vi "GetPoseAndTargeting.vi"() -> ()   [LabVIEW 2019]
uses:
  refnums.vi
  GRNF_GenericMotor.vi
  dsinstructions.vi
  sensors.vi
  autoninfo.vi
  dsdata.vi
panel:
  out "Y Position (in)":dbl=94.7
  out "X Position (in)":dbl=509.2
  out "Heading (deg)":dbl format="%#_13g"
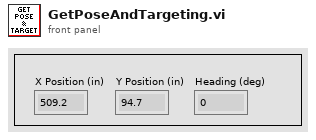
[diagram p1: front panel]
types:
  T1 = enum16{"Center", "North", "NorthWest", "West", "SouthWest", "South", "SouthEast", "East", "NorthEast"}
  T2 = typedef "WPI_MotorControlDeviceRef.ctl" = cluster{"DeviceStatus":errorcluster, "Type":T3, "PWM":cluster{"PWM Channel":T4, "DeadBand":T5}, "CAN":cluster{"Device Number":u8, "SetOutput VI Ref":variant, "GetOutput VI Ref":variant, "Enable VI Ref":variant, "Disable VI Ref":variant, "Data":variant}, "Invert":bool, "DIO PWM":cluster{"PWM \"Enable\" Channel":T4, "DIOChannel":T6, "PWM Rate":dbl}}
  T3 = typedef "WPI_MotorControlType.ctl" = enum16{"PWM", "CAN", "DIO PWM"}
  T4 = typedef "FPGA_DIOPWMChannel.ctl" = enum8{"PWM 0", "PWM 1", "PWM 2", "PWM 3", "PWM 4", "PWM 5", "PWM 6", "PWM 7", "PWM 8", "PWM 9", "PWM MXP 0", "PWM MXP 1", "PWM MXP 2", "PWM MXP 3", "PWM MXP 4", "PWM MXP 5", "PWM MXP 6", "PWM MXP 7", "PWM MXP 8", "PWM MXP 9", "Invalid"}
  T5 = typedef "WPI_PWMDeadband.ctl" = cluster{"Name":string, "maxPositivePwm":i32, "minPositivePwm":i32, "centerPwm":i32, "maxNegativePwm":i32, "minNegativePwm":i32, "angularRange":u16}
  T6 = typedef "FPGA_DIOChannel.ctl" = enum8{"DIO 0", "DIO 1", "DIO 2", "DIO 3", "DIO 4", "DIO 5", "DIO 6", "DIO 7", "DIO 8", "DIO 9", "DIO MXP 0", "DIO MXP 1", "DIO MXP 2", "DIO MXP 3", "DIO MXP 4", "DIO MXP 5", "DIO MXP 6", "DIO MXP 7", "DIO MXP 8", "DIO MXP 9", "DIO MXP 10", "DIO MXP 11", "DIO MXP 12", "DIO MXP 13", "DIO MXP 14", "DIO MXP 15", "SPI Port CS1", "SPI Port CS2", "SPI Port CS3", "SPI Port MISO", "SPI Port MOSI", "Invalid"}
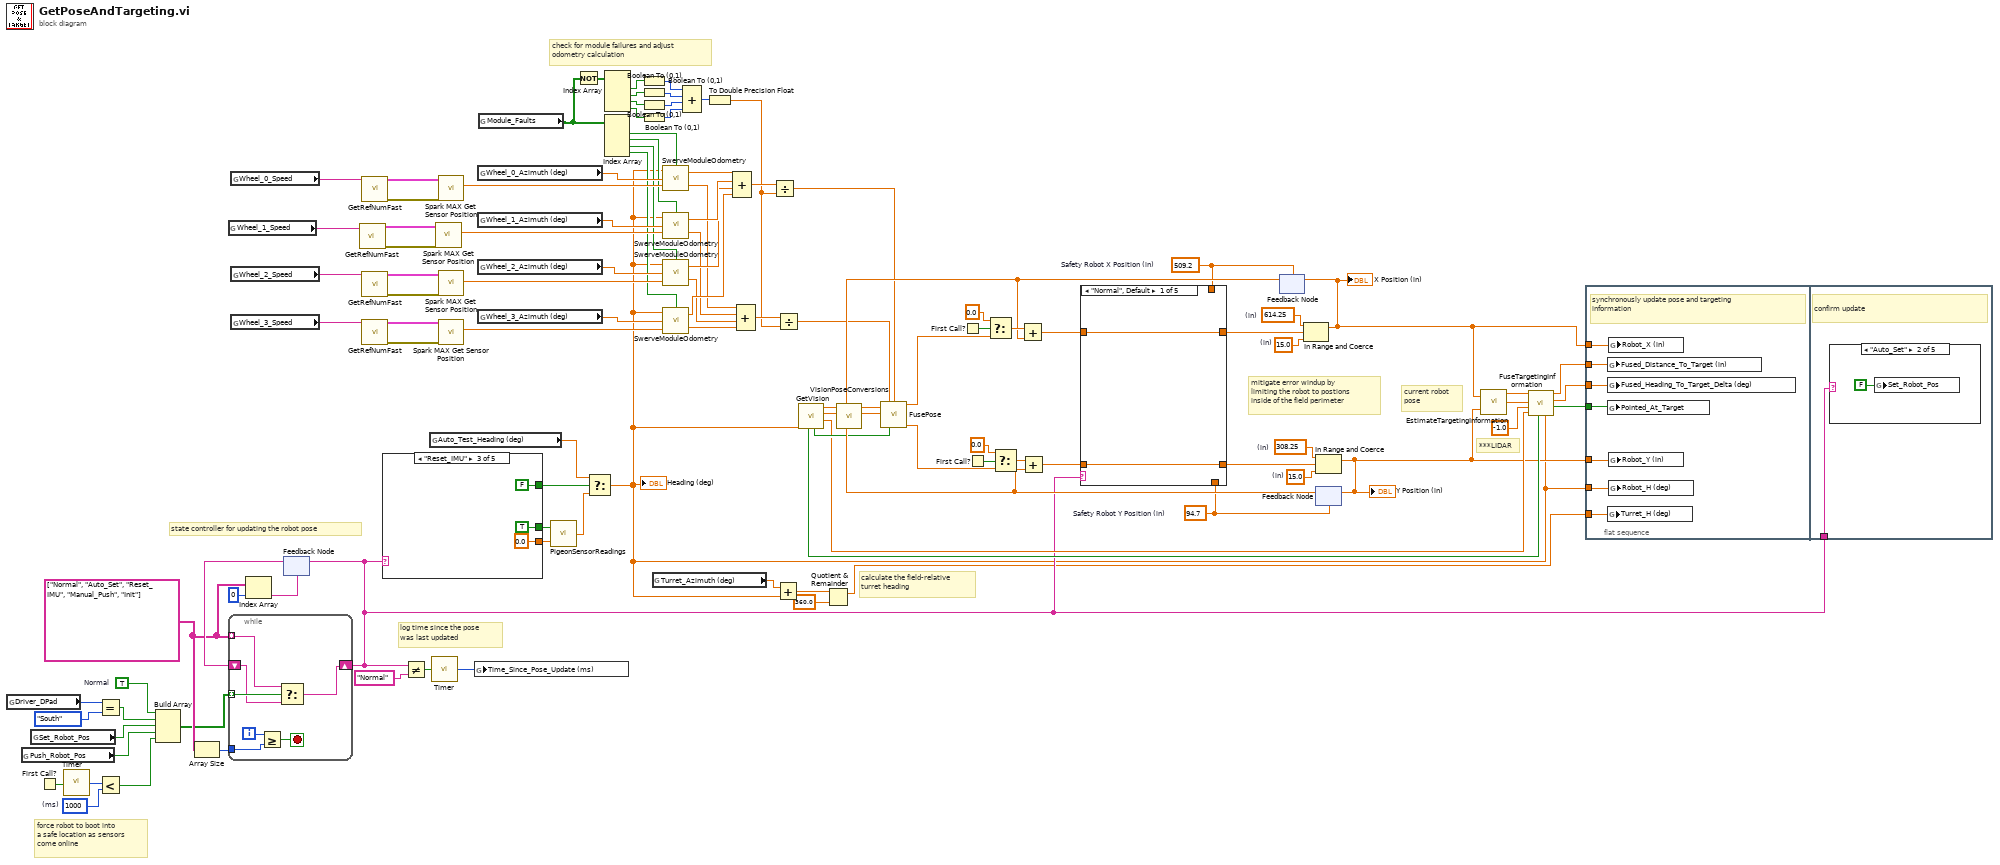
[diagram p0: block diagram]
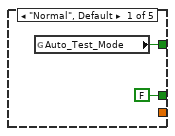
[diagram p6: hidden frame]
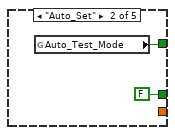
[diagram p7: hidden frame]
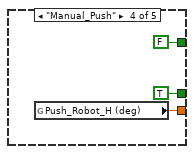
[diagram p8: hidden frame]
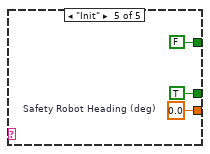
[diagram p9: hidden frame]
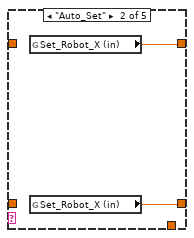
[diagram p10: hidden frame]
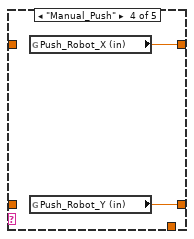
[diagram p12: hidden frame]
diagram:
  w2 = u32 1000  # (ms)
  w33 = string[] ["Normal", "Auto_Set", "Reset_IMU", "Manual_Push", "Init"] ("State Names")
  w32 = TRUE  # Normal
  w57 = 308.25  # (in)
  w58 = 15.0  # (in)
  w62 = 614.25  # (in)
  w63 = 15.0  # (in)
  w7 = 509.2  # Safety Robot X Position (in)
  w6 = 94.7  # Safety Robot Y Position (in)
  # "***LIDAR"
  # "force robot to boot into\na safe location as sensors\ncome online"
  # "calculate the field-relative\nturret heading"
  # "log time since the pose\nwas last updated"
  # "state controller for updating the robot pose"
  # "current robot\npose"
  # "mitigate error windup by\nlimiting the robot to postions\ninside of the field perimeter"
  # "check for module failures and adjust\nodometry calculation"
  n1 = global read "dsinstructions.vi" "Driver_DPad"() -> (w77:T1)
  n2 = global read "sensors.vi" "Push_Robot_Pos"() -> (w34:bool)
  n3 = global read "sensors.vi" "Set_Robot_Pos"() -> (w19:bool)
  n4 = First Call?() -> (First Call?: T/F=w5:bool)
  n5 = call "Timer.vi"("Reset Timer"=w5) -> ("Time (ms)"=w4:u32)
  n6 = Equal?(x=w77, y=T1."South") -> (x = y?=w31:bool)
  n7 = Less?(x=w4, y=w2) -> (x < y?=w3:bool)
  n8 = Build Array(w32, w31, w19, w34, w3) -> (w30:bool[])
  n9 = Array Size(array=w33) -> (size(s)=w35:i32)
  n10 = global read "refnums.vi" "Wheel_1_Speed"() -> (w70:string)
  n11 = global read "refnums.vi" "Wheel_0_Speed"() -> (w73:string)
  n12 = global read "refnums.vi" "Wheel_2_Speed"() -> (w67:string)
  n13 = global read "refnums.vi" "Wheel_3_Speed"() -> (w64:string)
  n14 = Index Array(array=w33, index=0) -> (element=w37:string)
  n15 = feedback #1(w37) -> (w36:string)
  n16 = while {
    tunnel: w30 -> [w120] mode=indexing
    tunnel: w33 -> [w118] mode=indexing
    shift-right: [w117] -> w17
    shift-left: w36 -> [w119]
    tunnel: w35 -> [w115]
    i -> [w116]
    stop <- w114 stop-if-true
    n17 = Greater Or Equal?(x=w116, y=w115) -> (x >= y?=w114:bool)
    n18 = Select(t=w118, s=w120, f=w119) -> (s? t:f=w117:string)
  }
  n19 = feedback-in #1(w17) -> ()
  n20 = call-poly "GetRefNumFast.vi"("RefNum Name"=w70) -> ("Error"=w71:errorcluster, "Device Reference"=w72:T2)  [unwired: 5 in]
  n21 = call-poly "GetRefNumFast.vi"("RefNum Name"=w73) -> ("Error"=w74:errorcluster, "Device Reference"=w75:T2)  [unwired: 5 in]
  n22 = call-poly "GetRefNumFast.vi"("RefNum Name"=w67) -> ("Error"=w68:errorcluster, "Device Reference"=w69:T2)  [unwired: 5 in]
  n23 = call-poly "GetRefNumFast.vi"("RefNum Name"=w64) -> ("Error"=w65:errorcluster, "Device Reference"=w66:T2)  [unwired: 5 in]
  n24 = case shown="\"Reset_IMU\"" w17 {
    tunnel: [_ _ 0.0 ("Push_Robot_H (deg)") w130 w131] -> w25
    tunnel: [FALSE FALSE TRUE TRUE TRUE] -> w24
    tunnel: [w121 w123 FALSE ("Auto_Test_Mode") FALSE ("Auto_Test_Mode") FALSE ("Auto_Test_Mode")] -> w8
    frame "Normal", Default {
      n25 = global read "dsdata.vi" "Auto_Test_Mode"() -> (w121:bool)
    }
    frame "Auto_Set" {
      n26 = global read "dsdata.vi" "Auto_Test_Mode"() -> (w123:bool)
    }
    frame "Reset_IMU" {
    }
    frame "Manual_Push" {
      n27 = global read "sensors.vi" "Push_Robot_H (deg)"() -> (w130:dbl)
    }
    frame "Init" {
      w131 = 0.0  # Safety Robot Heading (deg)
    }
  }
  n28 = Not Equal?(x=w17, y="Normal") -> (x != y?=w16:bool)
  n29 = global read "autoninfo.vi" "Auto_Test_Heading (deg)"() -> (w78:dbl)
  n30 = call "Timer.vi"("Reset Timer"=w16) -> ("Time (ms)"=w14:u32)
  n31 = call <vilib>:"Spark MAX Get Sensor Position.vi"("error in (no error)"=w71, "MotorControlDevRef in"=w72) -> ("Sensor Position"=w111:dbl)  [unwired: 6 in, 3 out]
  n32 = call <vilib>:"Spark MAX Get Sensor Position.vi"("error in (no error)"=w74, "MotorControlDevRef in"=w75) -> ("Sensor Position"=w113:dbl)  [unwired: 6 in, 3 out]
  n33 = call <vilib>:"Spark MAX Get Sensor Position.vi"("error in (no error)"=w68, "MotorControlDevRef in"=w69) -> ("Sensor Position"=w110:dbl)  [unwired: 6 in, 3 out]
  n34 = call <vilib>:"Spark MAX Get Sensor Position.vi"("error in (no error)"=w65, "MotorControlDevRef in"=w66) -> ("Sensor Position"=w96:dbl)  [unwired: 6 in, 3 out]
  n35 = global write "sensors.vi" "Time_Since_Pose_Update (ms)"(w14) -> ()
  n36 = global read "sensors.vi" "Wheel_0_Azimuth (deg)"() -> (w112:dbl)
  n37 = global read "sensors.vi" "Wheel_1_Azimuth (deg)"() -> (w109:dbl)
  n38 = global read "sensors.vi" "Wheel_2_Azimuth (deg)"() -> (w108:dbl)
  n39 = global read "sensors.vi" "Wheel_3_Azimuth (deg)"() -> (w97:dbl)
  n40 = global read "sensors.vi" "Module_Faults"() -> (w95:bool[])
  n41 = call "PigeonSensorReadings.vi"("Reset Yaw (deg)"=w25, "Reset Yaw"=w24) -> ("Yaw (deg)"=w79:dbl)
  n42 = Not(x=w95) -> (.not. x?=w94:bool[])
  n43 = Select(t=w78, s=w8, f=w79) -> (s? t:f=w10:dbl)
  "Heading (deg)" <- w10
  n44 = Index Array(array=w95) -> (element #1=w83:bool, element #2=w82:bool, element #3=w81:bool, element #4=w80:bool)  [unwired: 4 in]
  n45 = Index Array(array=w94) -> (element #1=w93:bool, element #2=w92:bool, element #3=w91:bool, element #4=w90:bool)  [unwired: 4 in]
  n46 = Boolean To (0,1)(Boolean=w93) -> (0, 1=w89:i16)
  n47 = Boolean To (0,1)(Boolean=w92) -> (0, 1=w88:i16)
  n48 = Boolean To (0,1)(Boolean=w91) -> (0, 1=w87:i16)
  n49 = Boolean To (0,1)(Boolean=w90) -> (0, 1=w86:i16)
  n50 = global read "sensors.vi" "Turret_Azimuth (deg)"() -> (w11:dbl)
  n51 = call "SwerveModuleOdometry.vi"("Module Fault"=w83, "Wheel Distance (native)"=w113, "Wheel Azimuth (deg)"=w112, "Robot Heading(deg)"=w10) -> ("Delta Y (in)"=w98:dbl, "Delta X (in)"=w107:dbl)
  n52 = call "SwerveModuleOdometry.vi"("Module Fault"=w82, "Wheel Distance (native)"=w111, "Wheel Azimuth (deg)"=w109, "Robot Heading(deg)"=w10) -> ("Delta Y (in)"=w99:dbl, "Delta X (in)"=w106:dbl)
  n53 = call "SwerveModuleOdometry.vi"("Module Fault"=w81, "Wheel Distance (native)"=w110, "Wheel Azimuth (deg)"=w108, "Robot Heading(deg)"=w10) -> ("Delta Y (in)"=w100:dbl, "Delta X (in)"=w105:dbl)
  n54 = call "SwerveModuleOdometry.vi"("Module Fault"=w80, "Wheel Distance (native)"=w96, "Wheel Azimuth (deg)"=w97, "Robot Heading(deg)"=w10) -> ("Delta Y (in)"=w101:dbl, "Delta X (in)"=w104:dbl)
  n55 = Compound Arithmetic op=ADD(w89, w88, w87, w86) -> (w85:i16)
  n56 = To Double Precision Float(number=w85) -> (double precision float=w84:dbl)
  n57 = Compound Arithmetic op=ADD(w107, w106, w105, w104) -> (w103:dbl)
  n58 = Compound Arithmetic op=ADD(w98, w99, w100, w101) -> (w102:dbl)
  n59 = Divide(x=w103, y=w84) -> (x/y=w47:dbl)
  n60 = Add(x=w11, y=w10) -> (x+y=w13:dbl)
  n61 = Divide(x=w102, y=w84) -> (x/y=w46:dbl)
  n62 = call "GetVision.vi"("Robot_H (deg)"=w10) -> ("LimeLight Raw Horizontal Offset (deg)"=w41:dbl, "LimeLight Raw X (in)"=w50:dbl, "LimeLight Raw Z (in)"=w51:dbl, "LimeLight Pose Valid"=w43:bool, "LimeLight Valid"=w42:bool)  [unwired: 6 in]
  n63 = Quotient & Remainder(x=w13, y=360.0) -> (x-y*floor(x/y)=w9:dbl)  [unwired: 1 out]
  n64 = First Call?() -> (First Call?: T/F=w60:bool)
  n65 = First Call?() -> (First Call?: T/F=w55:bool)
  n66 = feedback #2(w7) -> (w52:dbl)
  n67 = feedback #3(w6) -> (w53:dbl)
  n68 = call "VisionPoseConversions.vi"("Previous Y Estimate (in)"=w53, "Previous X Estimate (in)"=w52, "LimeLight Raw X (in)"=w50, "LimeLight Raw Z (in)"=w51) -> ("deltaY (in)"=w44:dbl, "deltaX (in)"=w45:dbl)  [unwired: 6 in]
  n69 = call "FusePose.vi"("LimeLight deltaX"=w45, "Odometry deltaY"=w46, "Odometry deltaX"=w47, "LimeLight deltaY"=w44, "LimeLight Pose Valid"=w43) -> ("Fused deltaX"=w49:dbl, "Fused deltaY"=w48:dbl)  [unwired: 9 in]
  n70 = Select(t=0.0, s=w60, f=w49) -> (s? t:f=w61:dbl)
  n71 = Select(t=0.0, s=w55, f=w48) -> (s? t:f=w56:dbl)
  n72 = Add(x=w61, y=w52) -> (x+y=w29:dbl)
  n73 = Add(x=w56, y=w53) -> (x+y=w27:dbl)
  n74 = case shown="\"Normal\", Default" w17 {
    tunnel: w29 -> [w135 _ w139 _ _]
    tunnel: [w135 w137 w139 w141 w143] -> w28
    tunnel: w27 -> [w134 _ w138 _ _]
    tunnel: [w134 w136 w138 w140 w142] -> w26
    tunnel: w7 -> [_ _ _ _ w143]
    tunnel: w6 -> [_ _ _ _ w142]
    frame "Normal", Default {
    }
    frame "Auto_Set" {
      n75 = global read "sensors.vi" "Set_Robot_X (in)"() -> (w137:dbl)
      n76 = global read "sensors.vi" "Set_Robot_X (in)"() -> (w136:dbl)
    }
    frame "Reset_IMU" {
    }
    frame "Manual_Push" {
      n77 = global read "sensors.vi" "Push_Robot_X (in)"() -> (w141:dbl)
      n78 = global read "sensors.vi" "Push_Robot_Y (in)"() -> (w140:dbl)
    }
    frame "Init" {
    }
  }
  n79 = In Range and Coerce(upper limit=w62, x=w28, lower limit=w63) -> (coerced(x)=w23:dbl)  [unwired: 1 out]
  "X Position (in)" <- w23
  n80 = feedback-in #2(w23) -> ()
  n81 = In Range and Coerce(upper limit=w57, x=w26, lower limit=w58) -> (coerced(x)=w22:dbl)  [unwired: 1 out]
  "Y Position (in)" <- w22
  n82 = feedback-in #3(w22) -> ()
  n83 = call "EstimateTargetingInformation.vi"("Robot X (in)"=w23, "Robot Y (in)"=w22) -> ("Estimated Distance to Target (in)"=w39:dbl, "Estimated Robot Heading to Target (deg)"=w40:dbl)  [unwired: 1 out]
  n84 = call "FuseTargetingInformation.vi"("Robot_H (deg)"=w10, "LimeLight Valid"=w42, "LimeLight Raw Horizontal Offset (deg)"=w41, "LIDAR Range (in)"=-1.0, "Estimated Heading to Target (deg)"=w40, "Estimated Distance to Target (in)"=w39) -> ("Pointed at Target"=w18:bool, "Fused Heading to Target Delta (deg)"=w20:dbl, "Fused Distance to Target (in)"=w21:dbl)  [unwired: 3 in]
  n85 = flat-sequence {
    tunnel: w23 -> [w150]
    tunnel: w22 -> [w149]
    tunnel: w21 -> [w148]
    tunnel: w20 -> [w147]
    tunnel: w18 -> [w146]
    tunnel: w10 -> [w145]
    tunnel: w9 -> [w144]
    tunnel: w17 -> [w151]
    frame #0 {
      # "synchronously update pose and targeting information"
      n86 = global write "sensors.vi" "Fused_Distance_To_Target (in)"(w148) -> ()
      n87 = global write "sensors.vi" "Fused_Heading_To_Target_Delta (deg)"(w147) -> ()
      n88 = global write "sensors.vi" "Pointed_At_Target"(w146) -> ()
      n89 = global write "sensors.vi" "Turret_H (deg)"(w144) -> ()
      n90 = global write "sensors.vi" "Robot_X (in)"(w150) -> ()
      n91 = global write "sensors.vi" "Robot_Y (in)"(w149) -> ()
      n92 = global write "sensors.vi" "Robot_H (deg)"(w145) -> ()
    }
    frame #1 {
      # "confirm update"
      n93 = case shown="\"Auto_Set\"" w151 {
        frame "Normal", Default {
        }
        frame "Auto_Set" {
          n94 = global write "sensors.vi" "Set_Robot_Pos"(FALSE ("Set_Robot_Pos")) -> ()
        }
        frame "Reset_IMU" {
        }
        frame "Manual_Push" {
        }
        frame "Init" {
        }
      }
    }
  }
